vi "Generate Signal.vi"(8 "error in":errorcluster, 9 "Offset":dbl format="%0.2p", 10 "Amplitude":dbl=1.0 format="%0.2p", 11 "Frequency":dbl=10.0 format="%0.2p") -> (0 "error out":errorcluster, 3 "Waveform Graph":waveform(dbl)(graph))   [LabVIEW 2017]
uses:
  <vilib>/measure/NI_MABase.lvlib
panel:
  # "Sine Wave Properties"
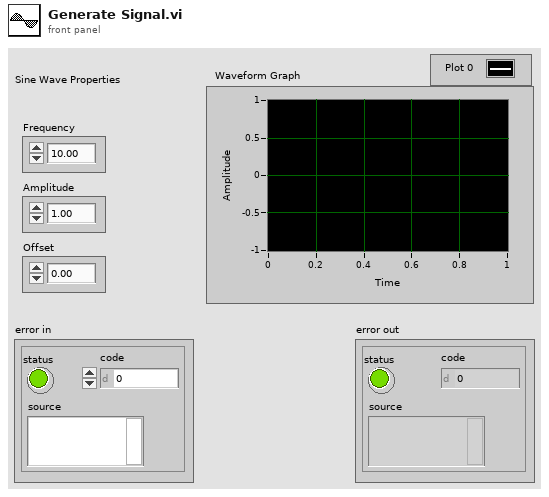
[diagram p1: front panel]
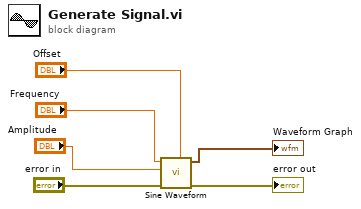
[diagram p0: block diagram]
diagram:
  n1 = call <vilib>:"Sine Waveform.vi"("offset"="Offset", "error in (no error)"="error in", "amplitude"="Amplitude", "frequency"="Frequency") -> ("error out"=→"error out":errorcluster, "signal out"=→"Waveform Graph":waveform(dbl))  [unwired: 6 in]
